vi "Write Sheet4 Data.vi"(0 "Cal Path":path, 9 "Dev Table 2":string[][](array[string]), 11 "Cal Point":i32) -> ()   [LabVIEW 2013]
uses:
  Type Defs/Excel Driver Operator Type Def.ctl
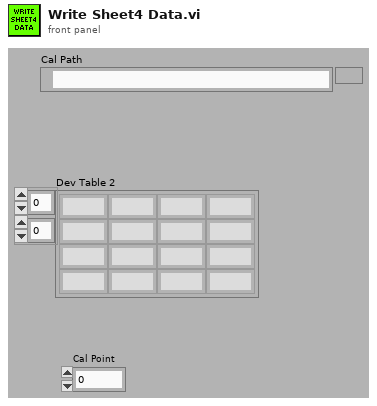
[diagram p1: front panel]
types:
  T1 = typedef "Excel Driver Operator Type Def.ctl" = enum16{"Open", "Close", "Search for String", "GetUsedRange", "Read Range", "Read Cell", "Set Range", "Set Cell"}
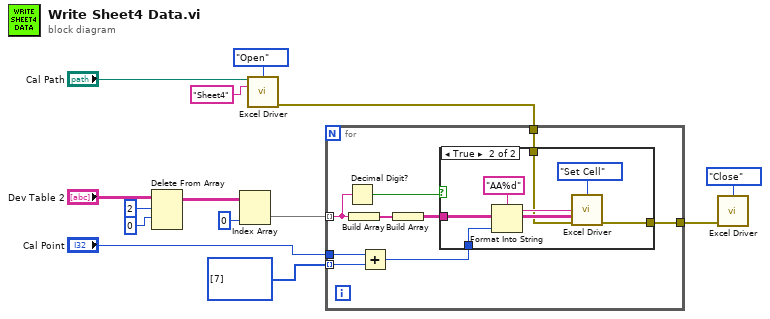
[diagram p0: block diagram]
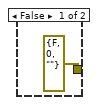
[diagram p2: hidden frame]
diagram:
  n1 = Delete From Array(array="Dev Table 2", length=2, index (row)=0) -> (array with subset deleted=w3:string[][])  [unwired: 1 in, 1 out]
  n2 = Index Array(array=w3, index (col)=0 ("disabled index (col)")) -> (element=w8:string[])  [unwired: 1 in]
  n3 = call "Excel Driver.vi"("Filename of Workbook"="Cal Path", "Operator"=Excel_Driver_Operator_Type_Def."Open", "WorkSheet Name"="Sheet4") -> ("error out"=w4:errorcluster)  [unwired: 10 in, 2 out]
  n4 = for {
    tunnel: w8 -> [w17] mode=indexing
    tunnel: [w21] -> w6
    tunnel: "Cal Point" -> [w20]
    tunnel: i32[] [7] -> [w19] mode=indexing
    tunnel: w4 -> [w15]
    n5 = Decimal Digit?(1:w17) -> (0:w16:bool)
    n6 = Build Array(w17) -> (w23:string[])
    n7 = Add(x=w20, y=w19) -> (x+y=w18:i32)
    n8 = Build Array(w23) -> (w22:string[][])
    n9 = case shown="True" w16 {
      tunnel: w22 -> [_ w30]
      tunnel: [errorcluster {"status"=FALSE, "code"=0, "source"=""} ("error out") w29] -> w21
      tunnel: w18 -> [_ w27]
      tunnel: w15 -> [_ w25]
      frame False {
      }
      frame True {
        n10 = Format Into String(format string="AA%d", w27) -> (resulting string=w28:string)  [unwired: 2 in, 1 out]
        n11 = call "Excel Driver.vi"("Operator"=Excel_Driver_Operator_Type_Def."Set Cell", "Range String\n(Or Search String)"=w28, "Cell Values INPUT"=w30, "error in (no error)"=w25) -> ("error out"=w29:errorcluster)  [unwired: 9 in, 2 out]
      }
    }
  }
  n12 = call "Excel Driver.vi"("Operator"=Excel_Driver_Operator_Type_Def."Close", "error in (no error)"=w6) -> ()  [unwired: 11 in, 3 out]
